vi "Identitiy.vi"(7 "QuWire in":refnum<class "QuWire.lvclass">) -> (8 "QuWire out":refnum<class "QuWire.lvclass">)   [LabVIEW 2020]
doc: "Identity Gate (I)\n\nNo-operation (No-Op). \nLeaves the quantum state unchanged. \nOften used as a placeholder."
uses:
  QuSim/QuWire/QuWire.lvclass
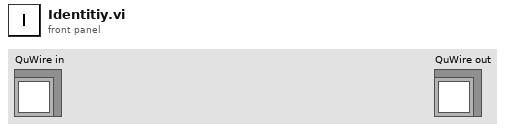
[diagram p1: front panel]
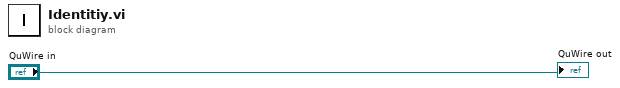
[diagram p0: block diagram]
diagram:
  "QuWire out" <- "QuWire in"
